vi "start_switch.vi"(2 "Switch heater time":dbl format="%#_13g") -> ()   [LabVIEW 2016]
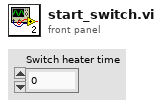
[diagram p1: front panel]
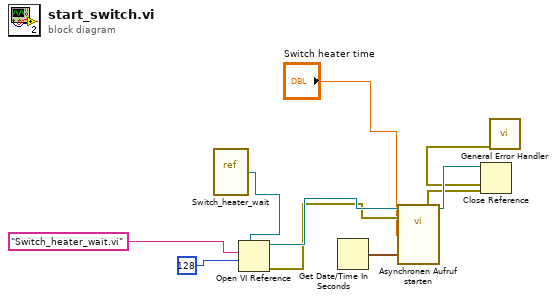
[diagram p0: block diagram]
diagram:
  n1 = vi-ref "Switch_heater_wait.vi"() -> (w2:refnum<vi>)
  n2 = Open VI Reference(type specifier VI Refnum (for type only)=w2, vi path="Switch_heater_wait.vi", options=128) -> (vi reference=w10:refnum<vi>, error out=w6:errorcluster)  [unwired: 3 in]
  n3 = Get Date/Time In Seconds() -> (seconds since 1Jan1904=w5:timestamp)
  n4 = call-by-ref "Asynchronen Aufruf starten"(reference=w10, error in=w6, "T-Start"=w5, "Switch waiting time"="Switch heater time") -> (reference out=w9:refnum<vi>, error out=w7:errorcluster)  [unwired: 1 in]
  n5 = Close Reference(reference=w9, error in (no error)=w7) -> (error out=w8:errorcluster)
  n6 = call <vilib>:"General Error Handler.vi"("error in (no error)"=w8) -> ()  [unwired: 10 in, 5 out]
